vi "Test Log No Warning Recorded Without Message.vi"(8 "error in (no error)":errorcluster, 11 "Test Case In":refnum<class "Logger Test.lvclass">) -> (0 "error out":errorcluster, 3 "Test Case Out":refnum<class "Logger Test.lvclass">)   [LabVIEW 2020, in "Logger Test.lvclass"]
uses:
  Logger Test.lvclass
  C:/Program Files (x86)/National Instruments/LabVIEW 2020/vi.lib/Astemes/LUnit/Test Case.lvclass
  source/Framework Test Suite/Mock Process/Mock Process.lvclass
  C:/Git/astemes-triarc-framework/source/Framework/Process/Process.lvclass
  C:/Git/astemes-triarc-framework/source/Framework/Logging/Logging.lvclass
  source/Framework Test Suite/Mock Log Handler/Mock Log Handler.lvclass
  source/Framework/Process/Process.lvclass/Process.ctl
  <vilib>/Astemes/LUnit/Test Case.lvclass/Test Case.ctl
  <vilib>/Astemes/LUnit/LUnit Assertion Result.lvclass/LUnit Assertion Result.ctl
  <vilib>/Astemes/LUnit/LUnit Test Case Result.lvclass/LUnit Test Case Result.ctl
  <vilib>/Astemes/LUnit/LUnit Method Result.lvclass/LUnit Method Result.ctl
  source/Framework/Process/Public/Lifecycle/Get Lifecycle State.vi
  source/Framework/Process/Protected/Messaging/Enqueue Message.vi
  <vilib>/Astemes/LUnit/Palette/Fail.vi
  <vilib>/Astemes/LUnit/Palette/Pass.vi
  <vilib>/Astemes/LUnit/Set Assertion Type.vi
  <vilib>/Utility/error.llb/Clear Errors.vi
  source/Framework/Process/Private/SubVIs/Handle Debug Data.vi
  <vilib>/Astemes/LUnit/Add test result.vi
  <vilib>/Astemes/LUnit/LUnit Write Passed.vi
  <vilib>/Astemes/LUnit/LUnit Write Message.vi
  <vilib>/Astemes/LUnit/LUnit Write Description.vi
  <vilib>/Astemes/LUnit/LUnit Write Assertion Type.vi
  source/Framework/Logging/Log Debug.vi
  <vilib>/AdvancedString/1D String Array to Delimited String.vi
  <vilib>/Utility/High Resolution Relative Seconds.vi
  <vilib>/Astemes/LUnit/LUnit Record Assertion Result.vi
  <vilib>/Astemes/LUnit/LUnit Aggregate Assertion Results.vi
  <vilib>/Astemes/LUnit/Assertion Result/LUnit Read Status.vi
  <vilib>/Astemes/LUnit/LUnit Read Message.vi
  <vilib>/Astemes/LUnit/LUnit Read Description.vi
  <vilib>/Astemes/LUnit/Method Result/LUnit Merge Status.vi
  <vilib>/Astemes/LUnit/LUnit Concatenate result strings.vi
  <vilib>/Utility/error.llb/Error Cluster From Error Code.vi
  source/Framework/Process/Public/Read Name.vi
  <vilib>/Astemes/LUnit/LUnit Assertion Result.lvclass
  source/Framework/Logging/Logging.lvclass
  Logger Test.lvclass/Logger Test.ctl
  source/Framework/Process/Process.lvclass
  <vilib>/Astemes/LUnit/Test Case.lvclass
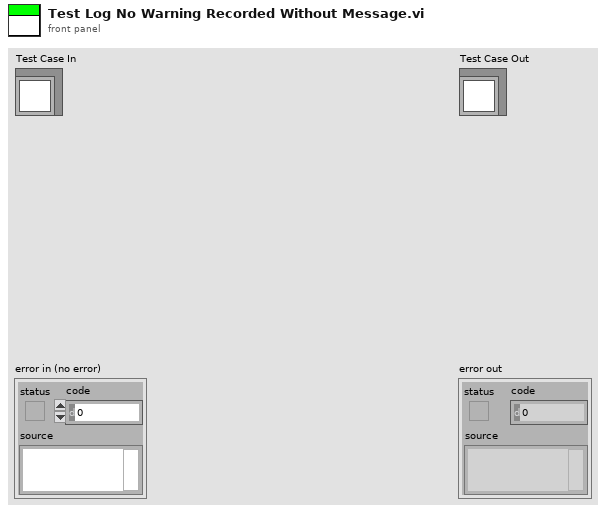
[diagram p1: front panel]
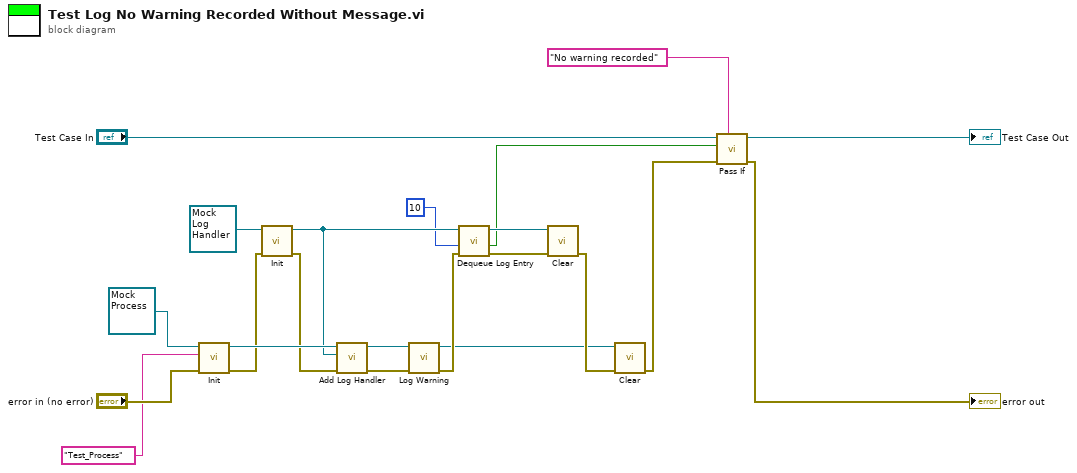
[diagram p0: block diagram]
diagram:
  n1 = call-dynamic "Init.vi"("error in (no error)"="error in (no error)", "Name"="Test_Process", "Mock Process In"=refnum<class "Mock Process.lvclass"> refnum) -> ("error out"=w14:errorcluster, "Mock Process Out"=w19:refnum<class "Mock Process.lvclass">)  [unwired: 7 in]
  n2 = call-dynamic "Init.vi"("error in (no error)"=w14, "Mock Log Handler In"=refnum<class "Mock Log Handler.lvclass"> refnum ("Mock Log Handler.lvclass")) -> ("error out"=w13:errorcluster, "Mock Log Handler Out"=w10:refnum<class "Mock Log Handler.lvclass">)  [unwired: 8 in]
  n3 = call "Add Log Handler.vi"("error in (no error)"=w13, "Log Handler"=w10, "Process In"=w19) -> ("error out"=w18:errorcluster, "Process Out"=w8:refnum<class "Mock Process.lvclass">)  [unwired: 7 in]
  n4 = call "Log Warning.vi"("error in (no error)"=w18, "Logging In"=w8) -> ("error out"=w7:errorcluster, "Logging Out"=w1:refnum<class "Mock Process.lvclass">)  [unwired: 8 in]
  n5 = call "Dequeue Log Entry.vi"("error in (no error)"=w7, "timeout in ms (-1)"=10, "Mock Log Handler in"=w10) -> ("error out"=w11:errorcluster, "timed out?"=w2:bool, "Mock Log Handler out"=w12:refnum<class "Mock Log Handler.lvclass">)  [unwired: 5 in, 1 out]
  n6 = call-dynamic "Clear.vi"("error in (no error)"=w11, "Mock Log Handler In"=w12) -> ("error out"=w6:errorcluster)  [unwired: 9 in]
  n7 = call-dynamic "Clear.vi"("error in (no error)"=w6, "Mock Process In"=w1) -> ("error out"=w4:errorcluster)  [unwired: 9 in]
  n8 = call <vilib>:"Pass If.vi"("Description"="No warning recorded", "error in (no error)"=w4, "Pass?"=w2, "LUnit Test Case In"="Test Case In") -> ("error out"=→"error out":errorcluster, "LUnit Test Case Out"=→"Test Case Out":refnum<class "Logger Test.lvclass">)  [unwired: 6 in]
